vi "Main.vi"() -> ()   [LabVIEW 2025]
doc: "This template is for the Queued Message Handler design pattern.\n\nThe Event Handling Loop generates messages based on user interface actions.\n\nThe Message Handling Loop processes messages generated by the Event Handling Loop, or by other messages. The messages are string values, so new messages can be added easily to the Message Cases case structure in the Message Handling Loop. Each message cluster can also provide an optional value for Message Data, which is a variant that can be converted to whatever message-specific data is required."
uses:
  Example 01/Support/AC parameters--cluster.ctl
  Example 01/Support/IR parameters--cluster.ctl
  controls/UI Data.ctl
  controls/AC Params--cluster.ctl
  controls/IR Params--cluster.ctl
  controls/Acquisition Data.ctl
  controls/Settings--cluster.ctl
  controls/Step--numeric.ctl
  support/Message Queue/Enqueue Message (Single).vi
  <vilib>/Utility/error.llb/Error Cluster From Error Code.vi
  support/Message Queue/Enqueue Message (Array).vi
  <vilib>/ErrorRing/Error Ring.xnode
  support/Message Queue/Message Queue.lvlib
  support/User Event - Stop/User Event - Stop.lvlib
  <instrlib>/Chrome 19025/Chrome 19025.lvlib
panel:
  in  "Set IR":bool
  in  "Set AC":bool
  out "Conn?":bool caption="Connected?"
  in  "VISA resource name":refnum<visa-resource-name>
  in  "Stop Test":bool
  in  "Start Test":bool
  out "IR Resistance":dbl(graph)
  out "AC Test Current":dbl(graph)
  in  "IR Parameters":T1={"Voltage Level [V]"=500, "Hi Limit [ohm]"=30000000000.0, "Test Time [s] "=8.0, "Dwell Time [s]"=4.4, "Lo Limit [ohm]"=2500000.0, "Ramp Time [s] "=1.1, "Fall Time [s]"=2.2} {"Voltage Level [V]" min=50 max=1000 step=1 format="%.3p"; "Hi Limit [ohm]" min=0.0 max=50000000000000.0 step=100000.0 format="%.1p"; "Test Time [s]" min=0.0 max=999.0 step=0.1 format="%.1p"; "Dwell Time [s]" min=0.0 max=999.0 step=0.1 format="%.1p"; "Lo Limit [ohm]" min=100000.0 max=50000000000000.0 step=100000.0 format="%.1p"; "Ramp Time [s]" min=0.0 max=999.0 step=0.1 format="%.1p"; "Fall Time [s]" min=0.0 max=999.0 step=0.1 format="%.1p"}
  in  "AC Parameters":T2={"Voltage Level [V] "=1500, "Hi Limit [A]"=0.005, "Test Time [s] "=8.0, "Lo Limit [A]"=0.0001, "ARC Limit [A]"=0.005, "Ramp Time [s] "=1.1, "Fall Time [s]"=2.2} {"Voltage Level [V]" min=50 max=5000 step=1 format="%.3p"; "Hi Limit [A]" min=0.0001 max=0.03 step=1e-07 format="%.2p"; "Test Time [s]" min=0.0 max=999.0 step=0.1 format="%.1p"; "Lo Limit [A]" min=0.0 max=0.03 step=1e-07 format="%.2p"; "ARC Limit [A]" min=0.0 max=15.0 format="%.1p"; "Ramp Time [s]" min=0.0 max=999.0 step=0.1 format="%.1p"; "Fall Time [s]" min=0.0 max=999.0 step=0.1 format="%.1p"}
  out "Messages":string
  in  "Exit":bool
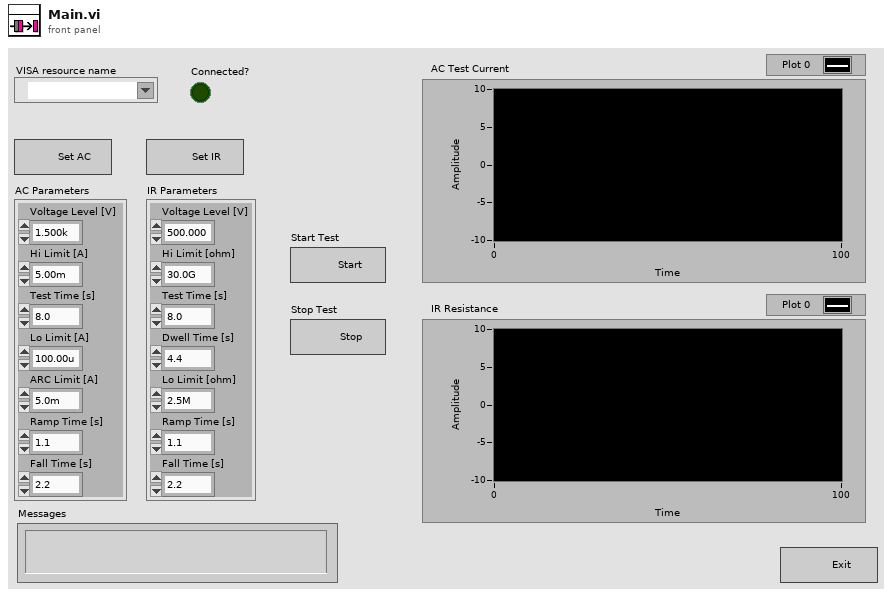
[diagram p1: front panel]
types:
  T1 = typedef "IR parameters--cluster.ctl" = cluster{"Voltage Level [V]":u16, "Hi Limit [ohm]":dbl, "Test Time [s] ":dbl, "Dwell Time [s]":dbl, "Lo Limit [ohm]":dbl, "Ramp Time [s] ":dbl, "Fall Time [s]":dbl}
  T2 = typedef "AC parameters--cluster.ctl" = cluster{"Voltage Level [V] ":u16, "Hi Limit [A]":dbl, "Test Time [s] ":dbl, "Lo Limit [A]":dbl, "ARC Limit [A]":dbl, "Ramp Time [s] ":dbl, "Fall Time [s]":dbl}
  T3 = typedef "UI Data.ctl" = cluster{"Connected?":bool, "Status":string, "Display Refnum":refnum<vi>, "Exit Refnum":refnum<vi>, "VISAName Refnum":refnum<vi>, "Settings":cluster{"VISA rsrc name":refnum<visa-resource-name>, "AC Parameters":T4, "IR Parameters":T5}}
  T4 = typedef "AC Params--cluster.ctl" = cluster{"Voltage Level [V] ":u16, "Hi Limit [A]":dbl, "Test Time [s] ":dbl, "Lo Limit [A]":dbl, "ARC Limit [A]":dbl, "Ramp Time [s] ":dbl, "Fall Time [s]":dbl}
  T5 = typedef "IR Params--cluster.ctl" = cluster{"Voltage Level [V]":u16, "Hi Limit [ohm]":dbl, "Test Time [s] ":dbl, "Dwell Time [s]":dbl, "Lo Limit [ohm]":dbl, "Ramp Time [s] ":dbl, "Fall Time [s]":dbl}
  T6 = typedef "Message Queue.lvlib/All Message Queues.ctl" = cluster{"UI":refnum<queue>, "Acquisition":refnum<queue>}
  T7 = cluster{"Baud Rate":u32, "Flow Control":u16, "Parity":u16, "Data Bits":u16}
  T8 = typedef "Settings--cluster.ctl" = cluster{"VISA rsrc name":refnum<visa-resource-name>, "AC Parameters":T4, "IR Parameters":T5}
  T9 = typedef "Acquisition Data.ctl" = cluster{"String <Replace Me>":string, "Numeric <Replace Me>":dbl, "Settings":cluster{"VISA rsrc name":refnum<visa-resource-name>, "AC Parameters":T4, "IR Parameters":T5}}
  T10 = typedef "Step--numeric.ctl" = u8
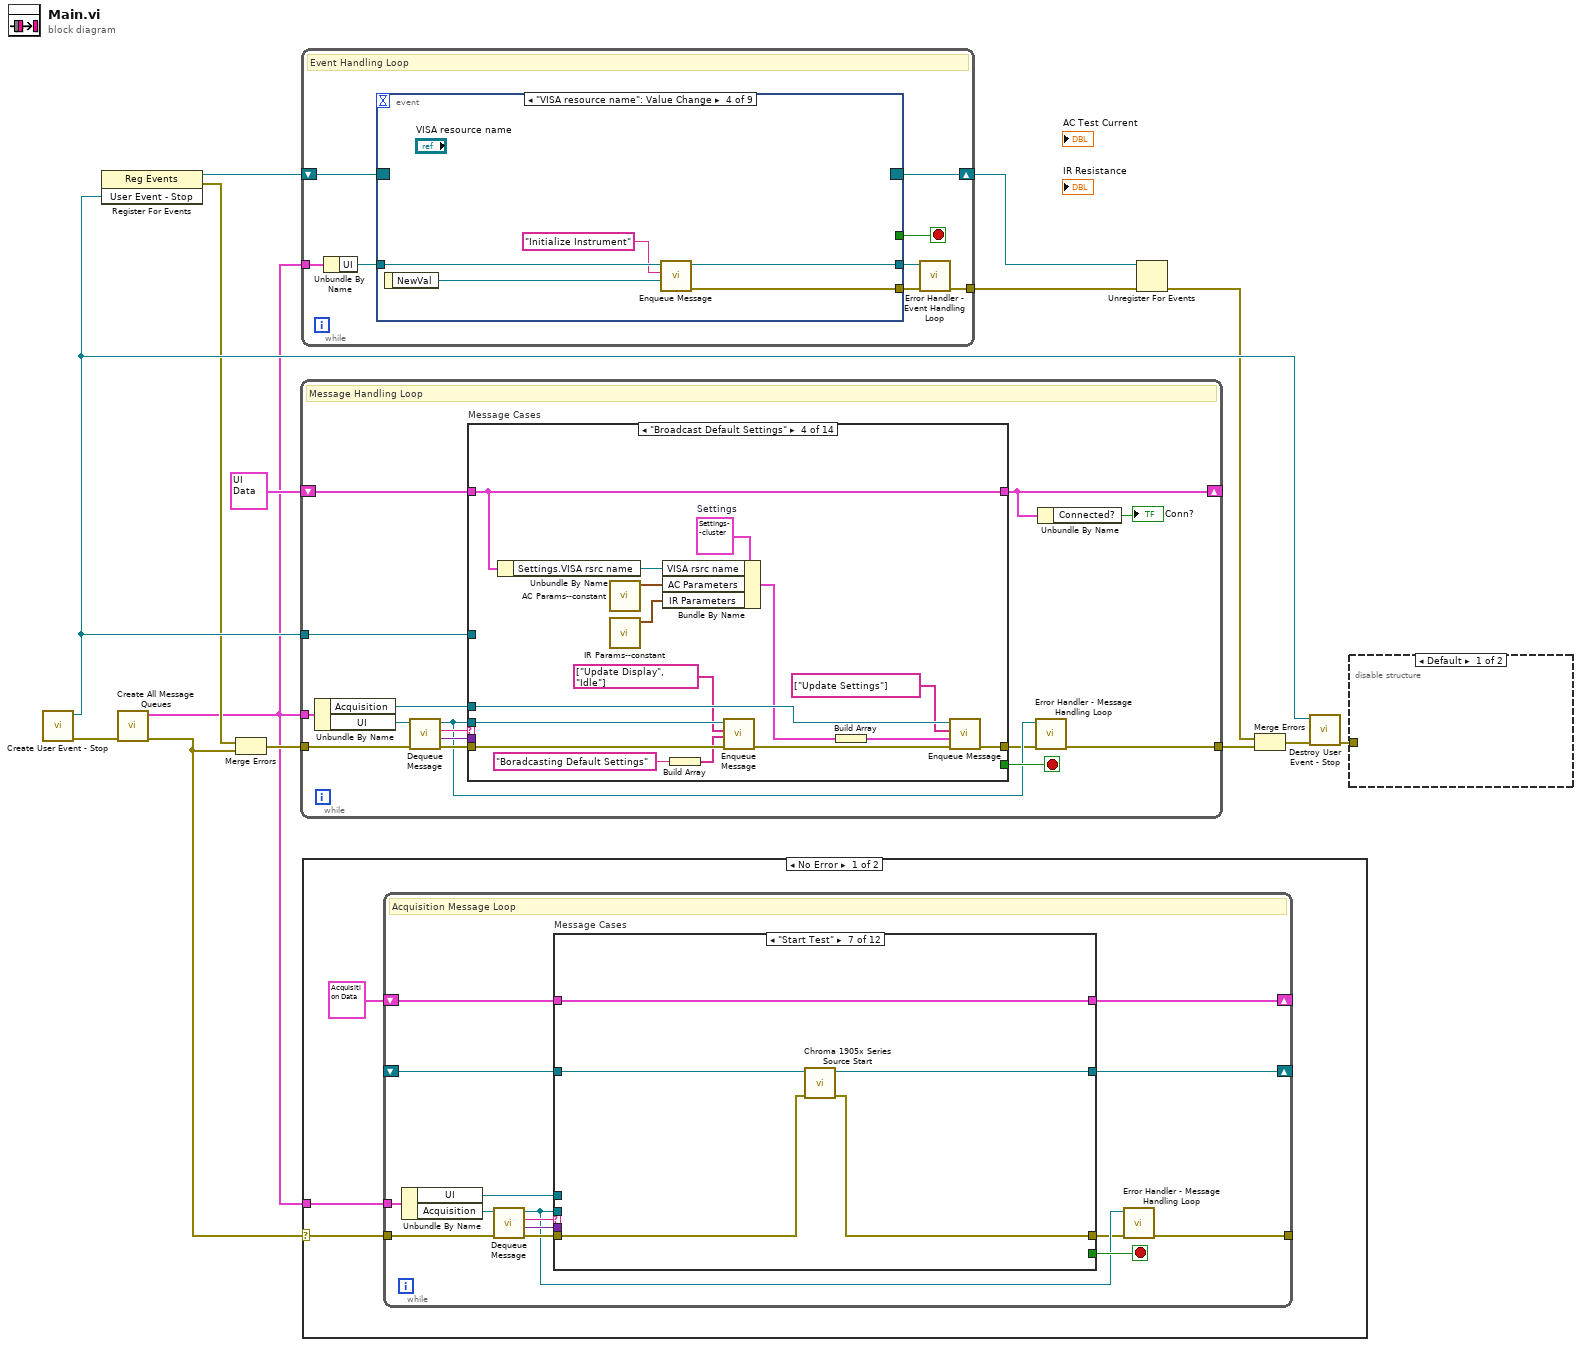
[diagram p0: block diagram]
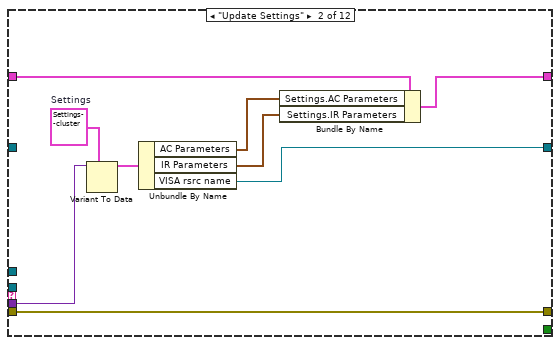
[diagram p3: hidden frame]
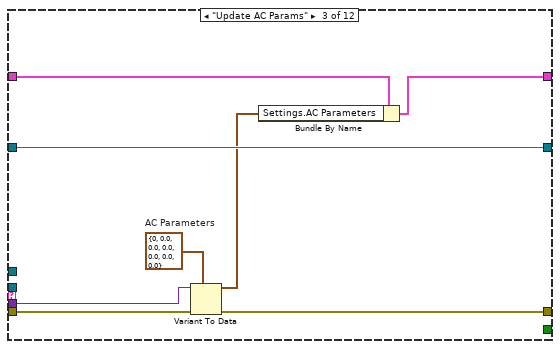
[diagram p4: hidden frame]
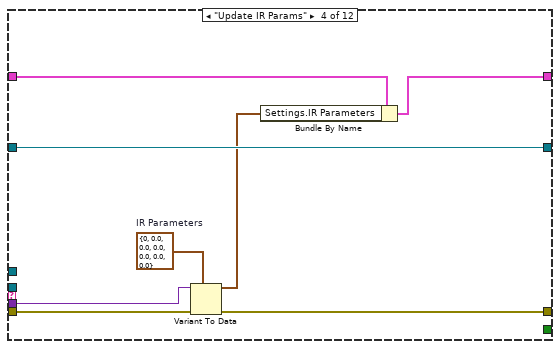
[diagram p5: hidden frame]
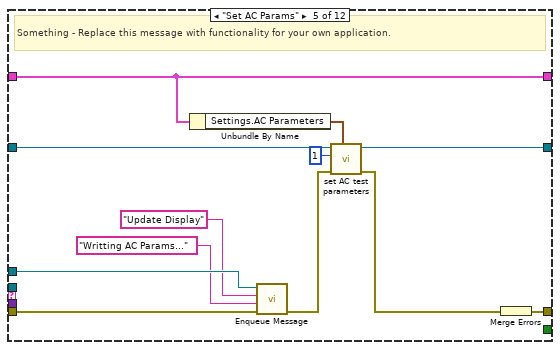
[diagram p6: hidden frame]
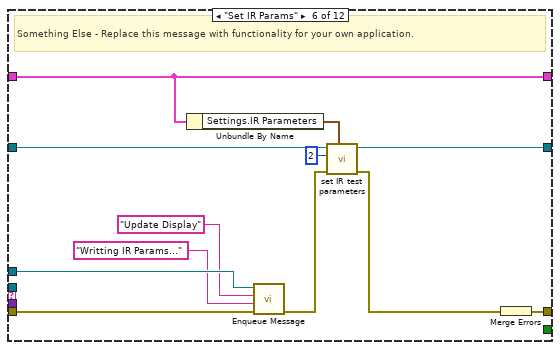
[diagram p7: hidden frame]
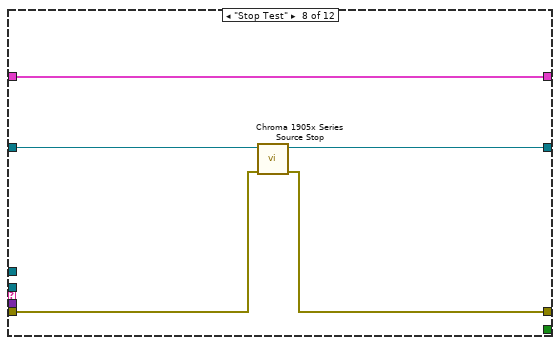
[diagram p8: hidden frame]
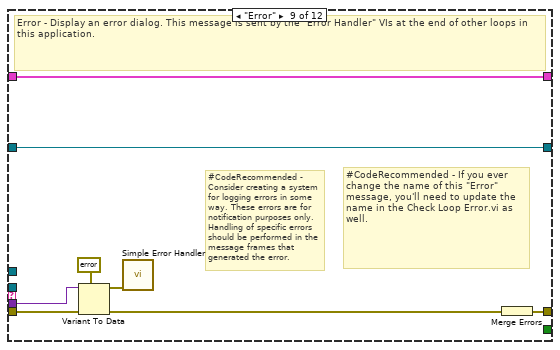
[diagram p9: hidden frame]
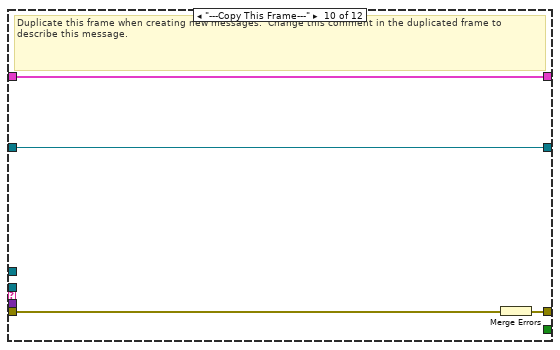
[diagram p10: hidden frame]
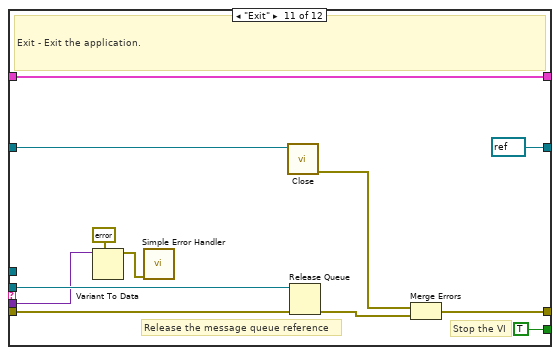
[diagram p11: hidden frame]
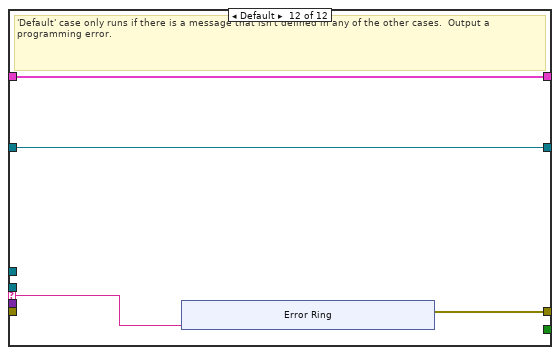
[diagram p12: hidden frame]
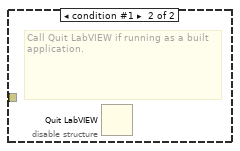
[diagram p14: hidden frame]
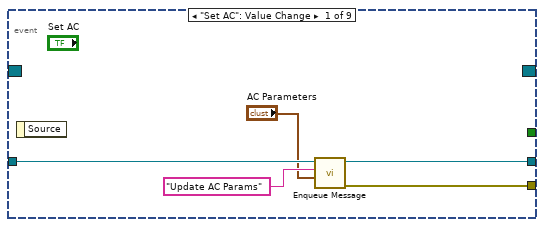
[diagram p15: hidden frame]
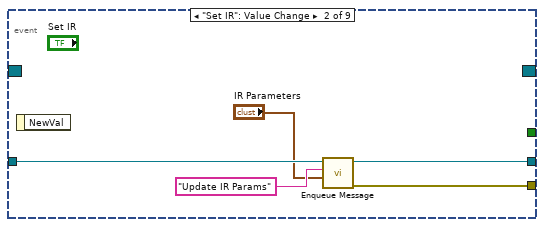
[diagram p16: hidden frame]
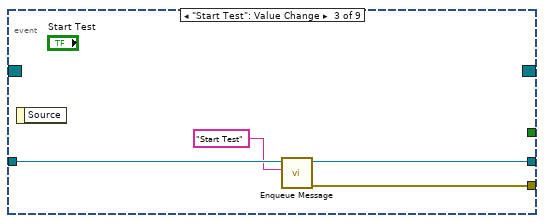
[diagram p17: hidden frame]
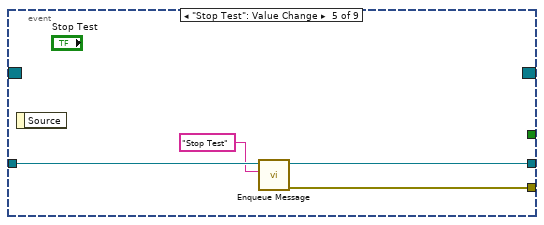
[diagram p18: hidden frame]
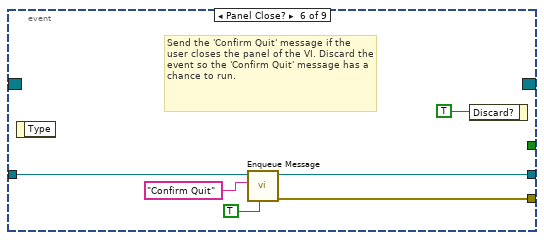
[diagram p19: hidden frame]
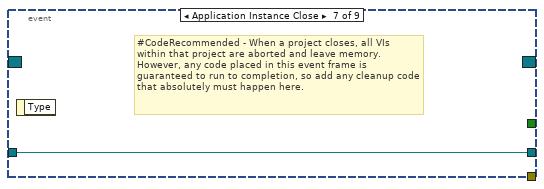
[diagram p20: hidden frame]
diagram:
  n1 = call "Create User Event - Stop.vi"() -> ("error out"=w11:errorcluster, "User Event - Stop"=w14:refnum<user-event>)  [unwired: 10 in]
  n2 = register-events(w14) -> (reference out=w4:refnum<event-registration>, error out=w13:errorcluster)  [unwired: 2 in]
  n3 = call "Create All Message Queues.vi"("error in (no error)"=w11) -> ("error out"=w2:errorcluster, "Message Queues out"=w1:T6)  [unwired: 9 in]
  n4 = Merge Errors(w13, w2) -> (w3:errorcluster)
  n5 = while {
    shift-right: [w17] -> _
    shift-left: T3 {"Connected?"=FALSE, "Status"="", "Display Refnum"=refnum, "Exit Refnum"=refnum, "VISAName Refnum"=refnum, "Settings"={"VISA rsrc name"="", "AC Parameters"={"Voltage Level [V] "=0, "Hi Limit [A]"=0.0, "Test Time [s] "=0.0, "Lo Limit [A]"=0.0, "ARC Limit [A]"=0.0, "Ramp Time [s] "=0.0, "Fall Time [s]"=0.0}, "IR Parameters"={"Voltage Level [V]"=0, "Hi Limit [ohm]"=0.0, "Test Time [s] "=0.0, "Dwell Time [s]"=0.0, "Lo Limit [ohm]"=0.0, "Ramp Time [s] "=0.0, "Fall Time [s]"=0.0}}} ("Data Cluster") -> [w29]
    tunnel: w14 -> [w27]
    tunnel: w3 -> [w26]
    tunnel: [w21] -> w12
    tunnel: w1 -> [w19]
    stop <- w28 stop-if-true
    # "Message Handling Loop"
    n6 = Unbundle By Name(w19) -> ("Acquisition"=w15:refnum<queue>, "UI"=w18:refnum<queue>)
    n7 = call "Dequeue Message.vi"("error in (no error)"=w26, "Message Queue"=w18) -> ("error out"=w25:errorcluster, "Message Data"=w23:variant, "Message"=w24:string, "dup Message Queue"=w22:refnum<queue>)  [unwired: 6 in]
    n8 = case "Message Cases" shown="\"Broadcast Default Settings\"" w24 {
      selector: w24 -> [_ _ _ _ _ _ _ _ _ _ _ _ _ w179]
      tunnel: w22 -> [w40 w45 w54 w80 w94 w105 w117 w124 _ _ w150 w161 w177 _]
      tunnel: w25 -> [w31 w44 w53 w82 w96 w114 w119 w132 w138 w147 w154 w156 w171 _]
      tunnel: [w39 w43 w55 w84 w100 w111 w122 w125 w139 w141 w152 w159 w174 w180] -> w20
      tunnel: w29 -> [w38 w47 w61 w78 w101 w112 w123 w130 w140 w146 w153 w160 w167 w181]
      tunnel: [w37 w46 w60 w78 w101 w112 w123 w130 w140 w146 w153 w160 w165 w181] -> w17
      tunnel: [_ _ _ _ _ _ _ _ _ _ _ _ TRUE _] -> w28
      tunnel: w23 -> [_ _ w50 _ w93 w106 _ _ w137 w145 _ _ w168 _]
      tunnel: w27 -> [_ _ _ _ _ _ _ _ _ _ _ _ w173 _]
      tunnel: w15 -> [_ _ _ w85 w99 w109 w121 w131 _ _ _ _ w178 _]
      frame "Initialize" {
        # "Initialize - All initialization work should take place in this message, since other loops can potentially enqueue messages that execute immediately after this one."
        n9 = control-ref of="VISA resource name"() -> (w30:refnum<vi>)
        n10 = control-ref of="Exit"() -> (w35:refnum<vi>)
        n11 = control-ref of="Display"() -> (w36:refnum<vi>)
        n12 = Bundle By Name(cluster=w38, "Display Refnum"=w36, "Exit Refnum"=w35, "VISAName Refnum"=w30) -> (w37:T3)
        n13 = Build Array("Initial Message" ("Initial Message")) -> (w32:string[])
        n14 = call-poly "Enqueue Message.vi"("error in (no error)"=w31, "Message Data Array"=w32, "Message Array"=string[] ["Update Display", "Get VISA Control Value"], "Message Queue"=w40) -> ("error out"=w39:errorcluster)  [unwired: 6 in, 1 out]
      }
      frame "Get VISA Control value" {
        n15 = Unbundle By Name(w47) -> ("VISAName Refnum"=w48:refnum<vi>)
        n16 = property class="VISAName"(reference=w48) -> ("Value"=w42:refnum<visa-resource-name>)  [unwired: 1 in, 2 out]
        n17 = Bundle By Name(cluster=w47, "Settings.VISA rsrc name"=w42) -> (w46:T3)
        n18 = call-poly "Enqueue Message.vi"("error in (no error)"=w44, "Message Data"=w42, "Message"="Initialize Instrument", "Message Queue"=w45) -> ("error out"=w43:errorcluster)  [unwired: 6 in, 1 out]
      }
      frame "Initialize Instrument" {
        n19 = call "Serial Params--constant.vi"() -> ("Serial Configuration"=w58:T7)  [unwired: 11 in]
        n20 = Variant To Data(error in=w53, type=refnum<visa-resource-name> refnum ("VISA resource name"), Variant=w50) -> (data=w49:refnum<visa-resource-name>, error out=w52:errorcluster)
        n21 = call <instrlib>:"Initialize.vi"("Serial Configuration"=w58, "error in (no error)"=w52, "Reset (True)"=FALSE, "VISA resource name"=w49) -> ("error out"=w56:errorcluster, "VISA resource name out"=w57:refnum<visa-resource-name>)  [unwired: 6 in]
        n22 = Not(x=w56) -> (.not. x?=w59:bool)
        n23 = case shown="No Error" w56 {
          selector: w56 -> [w66 w72]
          tunnel: [w65 w70] -> w55
          tunnel: w54 -> [w64 w69]
          frame No Error {
            n24 = call-poly "Enqueue Message.vi"("error in (no error)"=w66, "Message"="Broadcast Default Settings", "Message Queue"=w64) -> ("error out"=w65:errorcluster)  [unwired: 7 in, 1 out]
          }
          frame Error {
            n25 = call <vilib>:"Clear Errors.vi"("error in (no error)"=w72) -> ("error out"=w71:errorcluster)  [unwired: 5 in, 1 out]
            n26 = call-poly "Enqueue Message.vi"("error in (no error)"=w71, "Message Data"="Connection Error. Update VISA reference number to retry connection.", "Message"="Update Display", "Message Queue"=w69) -> ("error out"=w70:errorcluster)  [unwired: 6 in, 1 out]
          }
        }
        n27 = Bundle By Name(cluster=w61, "Settings.VISA rsrc name"=w57, "Connected?"=w59) -> (w60:T3)
      }
      frame "Broadcast Default Settings" {
        w86 = T8 {"VISA rsrc name"="", "AC Parameters"={"Voltage Level [V] "=0, "Hi Limit [A]"=0.0, "Test Time [s] "=0.0, "Lo Limit [A]"=0.0, "ARC Limit [A]"=0.0, "Ramp Time [s] "=0.0, "Fall Time [s]"=0.0}, "IR Parameters"={"Voltage Level [V]"=0, "Hi Limit [ohm]"=0.0, "Test Time [s] "=0.0, "Dwell Time [s]"=0.0, "Lo Limit [ohm]"=0.0, "Ramp Time [s] "=0.0, "Fall Time [s]"=0.0}}  # Settings
        n28 = Unbundle By Name(w78) -> ("Settings.VISA rsrc name"=w77:refnum<visa-resource-name>)
        n29 = call "AC Params--constant.vi"() -> ("AC Parameters"=w88:T4)  [unwired: 11 in]
        n30 = call "IR Params--constant.vi"() -> ("IR Parameters"=w87:T5)  [unwired: 11 in]
        n31 = Bundle By Name(cluster=w86, "VISA rsrc name"=w77, "AC Parameters"=w88, "IR Parameters"=w87) -> (w83:T8)
        n32 = Build Array("Boradcasting Default Settings") -> (w73:string[])
        n33 = call-poly "Enqueue Message.vi"("error in (no error)"=w82, "Message Data Array"=w73, "Message Array"=string[] ["Update Display", "Idle"], "Message Queue"=w80) -> ("error out"=w81:errorcluster)  [unwired: 6 in, 1 out]
        n34 = Build Array(w83) -> (w75:T8[])
        n35 = call-poly "Enqueue Message.vi"("error in (no error)"=w81, "Message Data Array"=w75, "Message Array"=string[] ["Update Settings"], "Message Queue"=w85) -> ("error out"=w84:errorcluster)  [unwired: 6 in, 1 out]
      }
      frame "Update AC Params" {
        # "Something - Replace this message with functionality for your own application."
        n36 = Build Array("Updating AC Params") -> (w89:string[])
        n37 = call-poly "Enqueue Message.vi"("error in (no error)"=w96, "Message Data Array"=w89, "Message Array"=string[] ["Update Display", "Idle"], "Message Queue"=w94) -> ("error out"=w95:errorcluster)  [unwired: 6 in, 1 out]
        n38 = Build Array(w93) -> (w92:variant[])
        n39 = call-poly "Enqueue Message.vi"("error in (no error)"=w95, "Message Data Array"=w92, "Message Array"=string[] ["Update AC Params", "Set AC Params"], "Message Queue"=w99) -> ("error out"=w98:errorcluster)  [unwired: 6 in, 1 out]
        n40 = Merge Errors(w98) -> (w100:errorcluster)
      }
      frame "Update IR Params" {
        # "Something Else - Replace this message with functionality for your own application."
        n41 = Build Array("Updating IR Params") -> (w102:string[])
        n42 = call-poly "Enqueue Message.vi"("error in (no error)"=w114, "Message Data Array"=w102, "Message Array"=string[] ["Update Display", "Idle"], "Message Queue"=w105) -> ("error out"=w113:errorcluster)  [unwired: 6 in, 1 out]
        n43 = Build Array(w106) -> (w108:variant[])
        n44 = call-poly "Enqueue Message.vi"("error in (no error)"=w113, "Message Data Array"=w108, "Message Array"=string[] ["Update IR Params", "Set IR Params"], "Message Queue"=w109) -> ("error out"=w110:errorcluster)  [unwired: 6 in, 1 out]
        n45 = Merge Errors(w110) -> (w111:errorcluster)
      }
      frame "Start Test" {
        n46 = call-poly "Enqueue Message.vi"("error in (no error)"=w119, "Message Data"="Starting Test..." ("Message"), "Message"="Update Display", "Message Queue"=w117) -> ("error out"=w118:errorcluster)  [unwired: 6 in, 1 out]
        n47 = call-poly "Enqueue Message.vi"("error in (no error)"=w118, "Message"="Start Test", "Message Queue"=w121) -> ("error out"=w122:errorcluster)  [unwired: 7 in, 1 out]
      }
      frame "Stop Test" {
        n48 = call-poly "Enqueue Message.vi"("error in (no error)"=w132, "Message Data"="Stopping Test..." ("Message"), "Message"="Update Display", "Message Queue"=w124) -> ("error out"=w128:errorcluster)  [unwired: 6 in, 1 out]
        n49 = call-poly "Enqueue Message.vi"("error in (no error)"=w128, "Message"="Stop Test", "Message Queue"=w131) -> ("error out"=w125:errorcluster)  [unwired: 7 in, 1 out]
      }
      frame "Update Display" {
        # "#CodeRecommended - If you wish to decouple the Message Handling Loop from your user interface, consider creating User Events (like the \"Stop\" event in this VI) to message the Event Handling Loop whenever the user interface needs updating."
        # "Update Display - Convert the message data to a string to display in the Data Display indicator."
        n50 = Variant To Data(error in=w138, type="", Variant=w137) -> (data=→"Messages":string, error out=w135:errorcluster)
        n51 = Wait (ms)(milliseconds to wait=u32 250) -> ()  [unwired: 1 out]
        n52 = Merge Errors(w135) -> (w139:errorcluster)
      }
      frame "Error" {
        # "#CodeRecommended - If you ever change the name of this \"Error\" message, you'll need to update the name in the Check Loop Error.vi as well."
        # "#CodeRecommended - Consider creating a system for logging errors in some way. These errors are for notification purposes only. Handling of specific errors should be performed in the message frames that generated the error."
        # "Error - Display an error dialog. This message is sent by the \"Error Handler\" VIs at the end of other loops in this application."
        n53 = Variant To Data(error in=w147, type=errorcluster {"status"=FALSE, "code"=0, "source"=""} ("error constant"), Variant=w145) -> (data=w143:errorcluster, error out=w142:errorcluster)
        n54 = call <vilib>:"Simple Error Handler.vi"("error in (no error)"=w143) -> ()  [unwired: 4 in, 5 out]
        n55 = Merge Errors(w142) -> (w141:errorcluster)
      }
      frame "Confirm Quit" {
        # "#CodeNeeded - If you want to provide an \"Are you sure\" dialog (or some other notification) before the application exits, place that code here. This message is typically sent from a Panel Close? event."
        # "Confirm Quit - Message that can confirm whether or not the user wants to exit the application."
        n56 = call-poly "Enqueue Message.vi"("Priority Message? (F)"=TRUE, "error in (no error)"=w154, "Message"="Exit", "Message Queue"=w150) -> ("error out"=w151:errorcluster)  [unwired: 6 in, 1 out]
        n57 = Merge Errors(w151) -> (w152:errorcluster)
      }
      frame "Idle" {
        n58 = call-poly "Enqueue Message.vi"("error in (no error)"=w156, "Message Data"="Ready...", "Message"="Update Display", "Message Queue"=w161) -> ("error out"=w155:errorcluster)  [unwired: 6 in, 1 out]
        n59 = Merge Errors(w155) -> (w159:errorcluster)
      }
      frame "Exit" {
        # "Stop the VI"
        # "Release the message queue reference"
        # "Exit - Exit the application."
        n60 = Variant To Data(type=errorcluster {"status"=FALSE, "code"=0, "source"=""} ("error constant"), Variant=w168) -> (data=w169:errorcluster)  [unwired: 1 in, 1 out]
        n61 = call <vilib>:"Simple Error Handler.vi"("error in (no error)"=w169) -> ()  [unwired: 4 in, 5 out]
        n62 = call-poly "Enqueue Message.vi"("Priority Message? (F)"=TRUE, "Message"="Exit", "Message Queue"=w178) -> ("error out"=w162:errorcluster)  [unwired: 7 in, 1 out]
        n63 = call "Fire User Event - Stop.vi"("User Event - Stop"=w173) -> ("error out"=w172:errorcluster)  [unwired: 10 in]
        n64 = Release Queue(queue=w177, error in (no error)=w171) -> (error out=w175:errorcluster)  [unwired: 1 in, 2 out]
        n65 = Bundle By Name(cluster=w167, "Connected?"=FALSE) -> (w165:T3)
        n66 = Merge Errors(w162, w172, w175) -> (w174:errorcluster)
      }
      frame Default {
        # "'Default' case only runs if there is a message that isn't defined in any of the other cases.  Output a programming error."
        n67 = xnode "Error Ring"("parameter 0"=w179) -> ("error out"=w180:errorcluster)
      }
    }
    n68 = call "Error Handler - Message Handling Loop.vi"("error in (no error)"=w20, "Message Queue"=w22) -> ("dup error in"=w21:errorcluster)  [unwired: 8 in, 1 out]
    n69 = Unbundle By Name(w17) -> ("Connected?"=→"Conn?":bool)
  }
  n70 = while {
    shift-right: [w195] -> w8
    shift-left: w4 -> [w196]
    tunnel: [w191] -> w5
    tunnel: w1 -> [w190]
    stop <- w193 stop-if-true
    # "Event Handling Loop"
    n71 = Unbundle By Name(w190) -> ("UI"=w189:refnum<queue>)
    n72 = event shown="[3] \"VISA resource name\": Value Change" {
      selector: w196 -> [_ _ _ _ _ _ _ _ _]
      dyn-events: [_ _ _ _ _ _ _ _ _] -> w195
      timeout: _ -> [_ _ _ _ _ _ _ _ _]
      tunnel: [_ _ _ _ _ _ _ _ TRUE ("Discard?")] -> w193
      tunnel: w189 -> [w201 w206 w210 w215 w219 w224 w226 w231 w234]
      tunnel: [w198 w203 w208 w213 w217 w223 _ w230 _] -> w194
      tunnel: [w200 w205 w209 w214 w218 w222 w226 w229 w234] -> w192
      event "Set AC": Value Change {
        n73 = event-data() -> ()  [unwired: 1 in, 1 out]
        n74 = call-poly "Enqueue Message.vi"("Message Data"="AC Parameters", "Message"="Update AC Params", "Message Queue"=w201) -> ("error out"=w198:errorcluster, "dup Message Queue"=w200:refnum<queue>)  [unwired: 7 in]
      }
      event "Set IR": Value Change {
        n75 = event-data() -> ()  [unwired: 1 in, 1 out]
        n76 = call-poly "Enqueue Message.vi"("Message Data"="IR Parameters", "Message"="Update IR Params", "Message Queue"=w206) -> ("error out"=w203:errorcluster, "dup Message Queue"=w205:refnum<queue>)  [unwired: 7 in]
      }
      event "Start Test": Value Change {
        n77 = event-data() -> ()  [unwired: 1 in, 1 out]
        n78 = call-poly "Enqueue Message.vi"("Message"="Start Test", "Message Queue"=w210) -> ("error out"=w208:errorcluster, "dup Message Queue"=w209:refnum<queue>)  [unwired: 8 in]
      }
      event "VISA resource name": Value Change {
        n79 = event-data() -> ("NewVal"=w212:refnum<visa-resource-name>)  [unwired: 1 in]
        n80 = call-poly "Enqueue Message.vi"("Message Data"=w212, "Message"="Initialize Instrument", "Message Queue"=w215) -> ("error out"=w213:errorcluster, "dup Message Queue"=w214:refnum<queue>)  [unwired: 7 in]
      }
      event "Stop Test": Value Change {
        n81 = event-data() -> ()  [unwired: 1 in, 1 out]
        n82 = call-poly "Enqueue Message.vi"("Message"="Stop Test", "Message Queue"=w219) -> ("error out"=w217:errorcluster, "dup Message Queue"=w218:refnum<queue>)  [unwired: 8 in]
      }
      event Panel Close? {
        # "Send the 'Confirm Quit' message if the user closes the panel of the VI. Discard the event so the 'Confirm Quit' message has a chance to run."
        n83 = event-data() -> ()  [unwired: 1 in, 1 out]
        n84 = call-poly "Enqueue Message.vi"("Priority Message? (F)"=TRUE, "Message"="Confirm Quit", "Message Queue"=w224) -> ("error out"=w223:errorcluster, "dup Message Queue"=w222:refnum<queue>)  [unwired: 7 in]
        n85 = event-data("Discard?"=TRUE) -> ()  [unwired: 1 in, 1 out]
      }
      event Application Instance Close {
        # "#CodeRecommended - When a project closes, all VIs within that project are aborted and leave memory. However, any code placed in this event frame is guaranteed to run to completion, so add any cleanup code that absolutely must happen here."
        n86 = event-data() -> ()  [unwired: 1 in, 1 out]
      }
      event "Exit": Value Change {
        n87 = event-data() -> ()  [unwired: 1 in, 1 out]
        n88 = call-poly "Enqueue Message.vi"("Priority Message? (F)"=TRUE, "Message"="Exit", "Message Queue"=w231) -> ("error out"=w230:errorcluster, "dup Message Queue"=w229:refnum<queue>)  [unwired: 7 in]
      }
      event User Event {
        # "The Message Handling Loop processed an \"Exit\" message, which fired this event to stop the Event Handling Loop."
        n89 = event-data() -> ()  [unwired: 1 in, 1 out]
        n90 = local write "Messages"("\"Exit\" button pressed" ("VI Stopped")) -> ()
      }
    }
    n91 = call "Error Handler - Event Handling Loop.vi"("error in (no error)"=w194, "Message Queue"=w192) -> ("dup error in"=w191:errorcluster)  [unwired: 8 in, 1 out]
  }
  n92 = case shown="No Error" w2 {
    selector: w2 -> [w237 _]
    tunnel: w1 -> [w236 _]
    frame No Error {
      n93 = while {
        shift-right: [w243] -> _
        shift-left: T9 {"String <Replace Me>"="", "Numeric <Replace Me>"=0.0, "Settings"={"VISA rsrc name"="", "AC Parameters"={"Voltage Level [V] "=0, "Hi Limit [A]"=0.0, "Test Time [s] "=0.0, "Lo Limit [A]"=0.0, "ARC Limit [A]"=0.0, "Ramp Time [s] "=0.0, "Fall Time [s]"=0.0}, "IR Parameters"={"Voltage Level [V]"=0, "Hi Limit [ohm]"=0.0, "Test Time [s] "=0.0, "Dwell Time [s]"=0.0, "Lo Limit [ohm]"=0.0, "Ramp Time [s] "=0.0, "Fall Time [s]"=0.0}}} ("Acq Data") -> [w252]
        tunnel: w237 -> [w250]
        tunnel: [w245] -> _
        tunnel: w236 -> [w242]
        shift-right: [w240] -> _
        shift-left: _ -> [w239]
        stop <- w251 stop-if-true
        # "Acquisition Message Loop"
        n94 = Unbundle By Name(w242) -> ("UI"=w238:refnum<queue>, "Acquisition"=w241:refnum<queue>)
        n95 = call "Dequeue Message.vi"("error in (no error)"=w250, "Message Queue"=w241) -> ("error out"=w249:errorcluster, "Message Data"=w247:variant, "Message"=w248:string, "dup Message Queue"=w246:refnum<queue>)  [unwired: 6 in]
        n96 = case "Message Cases" shown="\"Start Test\"" w248 {
          selector: w248 -> [_ _ _ _ _ _ _ _ _ _ _ w340]
          tunnel: w246 -> [_ _ _ _ _ _ _ _ _ _ w338 _]
          tunnel: w249 -> [w253 w256 w269 w277 w283 w295 w306 w312 w322 w326 w334 _]
          tunnel: [w253 w256 w268 w276 w291 w303 w305 w311 w316 w324 w335 w341] -> w244
          tunnel: w252 -> [w254 w260 w271 w279 w288 w299 w309 w314 w321 w325 w327 w342]
          tunnel: [w254 w257 w270 w278 w288 w299 w309 w314 w321 w325 w327 w342] -> w243
          tunnel: [_ _ _ _ _ _ _ _ _ _ TRUE _] -> w251
          tunnel: w247 -> [_ w263 w267 w275 _ _ _ _ w320 _ w331 _]
          tunnel: [w255 w261 w272 w280 w290 w302 w307 w313 w315 w323 refnum<visa-resource-name> refnum ("VISA resource name") w339] -> w240
          tunnel: w239 -> [w255 _ w272 w280 w286 w298 w308 w310 w315 w323 w329 w339]
          tunnel: w238 -> [_ _ _ _ w292 w304 _ _ _ _ _ _]
          frame "Initialize" {
            # "Initialize - All initialization work should take place in this message, since other loops can potentially enqueue messages that execute immediately after this one."
          }
          frame "Update Settings" {
            w264 = T8 {"VISA rsrc name"="", "AC Parameters"={"Voltage Level [V] "=0, "Hi Limit [A]"=0.0, "Test Time [s] "=0.0, "Lo Limit [A]"=0.0, "ARC Limit [A]"=0.0, "Ramp Time [s] "=0.0, "Fall Time [s]"=0.0}, "IR Parameters"={"Voltage Level [V]"=0, "Hi Limit [ohm]"=0.0, "Test Time [s] "=0.0, "Dwell Time [s]"=0.0, "Lo Limit [ohm]"=0.0, "Ramp Time [s] "=0.0, "Fall Time [s]"=0.0}}  # Settings
            n97 = Variant To Data(type=w264, Variant=w263) -> (data=w262:T8)  [unwired: 1 in, 1 out]
            n98 = Unbundle By Name(w262) -> ("AC Parameters"=w259:T4, "IR Parameters"=w258:T5, "VISA rsrc name"=w261:refnum<visa-resource-name>)
            n99 = Bundle By Name(cluster=w260, "Settings.AC Parameters"=w259, "Settings.IR Parameters"=w258) -> (w257:T9)
          }
          frame "Update AC Params" {
            w266 = T4 {"Voltage Level [V] "=0, "Hi Limit [A]"=0.0, "Test Time [s] "=0.0, "Lo Limit [A]"=0.0, "ARC Limit [A]"=0.0, "Ramp Time [s] "=0.0, "Fall Time [s]"=0.0}  # AC Parameters
            n100 = Variant To Data(error in=w269, type=w266, Variant=w267) -> (data=w265:T4, error out=w268:errorcluster)
            n101 = Bundle By Name(cluster=w271, "Settings.AC Parameters"=w265) -> (w270:T9)
          }
          frame "Update IR Params" {
            w274 = T5 {"Voltage Level [V]"=0, "Hi Limit [ohm]"=0.0, "Test Time [s] "=0.0, "Dwell Time [s]"=0.0, "Lo Limit [ohm]"=0.0, "Ramp Time [s] "=0.0, "Fall Time [s]"=0.0}  # IR Parameters
            n102 = Variant To Data(error in=w277, type=w274, Variant=w275) -> (data=w273:T5, error out=w276:errorcluster)
            n103 = Bundle By Name(cluster=w279, "Settings.IR Parameters"=w273) -> (w278:T9)
          }
          frame "Set AC Params" {
            # "Something - Replace this message with functionality for your own application."
            n104 = Unbundle By Name(w288) -> ("Settings.AC Parameters"=w287:T4)
            n105 = call-poly "Enqueue Message.vi"("error in (no error)"=w283, "Message Data"="Writting AC Params...", "Message"="Update Display", "Message Queue"=w292) -> ("error out"=w284:errorcluster)  [unwired: 6 in, 1 out]
            n106 = call "set AC test parameters.vi"("AC Parameters"=w287, "error in (no error)"=w284, "Step"=T10 1, "VISA Refnum in"=w286) -> ("error out"=w289:errorcluster, "VISA Refnum out"=w290:refnum<visa-resource-name>)  [unwired: 6 in]
            n107 = Merge Errors(w289) -> (w291:errorcluster)
          }
          frame "Set IR Params" {
            # "Something Else - Replace this message with functionality for your own application."
            n108 = Unbundle By Name(w299) -> ("Settings.IR Parameters"=w300:T5)
            n109 = call-poly "Enqueue Message.vi"("error in (no error)"=w295, "Message Data"="Writting IR Params...", "Message"="Update Display", "Message Queue"=w304) -> ("error out"=w294:errorcluster)  [unwired: 6 in, 1 out]
            n110 = call "set IR test parameters.vi"("IR Parameters"=w300, "error in (no error)"=w294, "Step"=T10 2, "VISA Refnum in"=w298) -> ("error out"=w301:errorcluster, "VISA Refnum out"=w302:refnum<visa-resource-name>)  [unwired: 6 in]
            n111 = Merge Errors(w301) -> (w303:errorcluster)
          }
          frame "Start Test" {
            n112 = call "Chroma 1905x Series Source Start.vi"("error in (no error)"=w306, "VISA resource name"=w308) -> ("error out"=w305:errorcluster, "VISA resource name out"=w307:refnum<visa-resource-name>)  [unwired: 8 in]
          }
          frame "Stop Test" {
            n113 = call "Chroma 1905x Series Source Stop.vi"("error in (no error)"=w312, "VISA resource name"=w310) -> ("error out"=w311:errorcluster, "VISA resource name out"=w313:refnum<visa-resource-name>)  [unwired: 8 in]
          }
          frame "Error" {
            # "#CodeRecommended - If you ever change the name of this \"Error\" message, you'll need to update the name in the Check Loop Error.vi as well."
            # "#CodeRecommended - Consider creating a system for logging errors in some way. These errors are for notification purposes only. Handling of specific errors should be performed in the message frames that generated the error."
            # "Error - Display an error dialog. This message is sent by the \"Error Handler\" VIs at the end of other loops in this application."
            n114 = Variant To Data(error in=w322, type=errorcluster {"status"=FALSE, "code"=0, "source"=""} ("error constant"), Variant=w320) -> (data=w318:errorcluster, error out=w317:errorcluster)
            n115 = call <vilib>:"Simple Error Handler.vi"("error in (no error)"=w318) -> ()  [unwired: 4 in, 5 out]
            n116 = Merge Errors(w317) -> (w316:errorcluster)
          }
          frame "---Copy This Frame---" {
            # "Duplicate this frame when creating new messages.  Change this comment in the duplicated frame to describe this message."
            n117 = Merge Errors(w326) -> (w324:errorcluster)
          }
          frame "Exit" {
            # "Stop the VI"
            # "Release the message queue reference"
            # "Exit - Exit the application."
            n118 = Variant To Data(type=errorcluster {"status"=FALSE, "code"=0, "source"=""} ("error constant"), Variant=w331) -> (data=w332:errorcluster)  [unwired: 1 in, 1 out]
            n119 = call <vilib>:"Simple Error Handler.vi"("error in (no error)"=w332) -> ()  [unwired: 4 in, 5 out]
            n120 = call <instrlib>:"Close.vi"("VISA resource name"=w329) -> ("error out"=w328:errorcluster)  [unwired: 10 in]
            n121 = Release Queue(queue=w338, error in (no error)=w334) -> (error out=w336:errorcluster)  [unwired: 1 in, 2 out]
            n122 = Merge Errors(w328, w336) -> (w335:errorcluster)
          }
          frame Default {
            # "'Default' case only runs if there is a message that isn't defined in any of the other cases.  Output a programming error."
            n123 = xnode "Error Ring"("parameter 0"=w340) -> ("error out"=w341:errorcluster)
          }
        }
        n124 = call "Error Handler - Message Handling Loop.vi"("error in (no error)"=w244, "Message Queue"=w246) -> ("dup error in"=w245:errorcluster)  [unwired: 8 in, 1 out]
      }
    }
    frame Error {
    }
  }
  n125 = Unregister For Events(event registration refnum=w8, error in=w5) -> (error out=w9:errorcluster)
  n126 = Merge Errors(w9, w12) -> (w10:errorcluster)
  n127 = call "Destroy User Event - Stop.vi"("error in (no error)"=w10, "User Event - Stop"=w14) -> ("error out"=w6:errorcluster)  [unwired: 9 in]
  n128 = disable-structure shown="Default" {
    disable-tunnel: w6 -> [_ _]
    frame condition #0 (active) {
    }
    frame condition #1 {
      # "Call Quit LabVIEW if running as a built application."
      n129 = Quit LabVIEW() -> ()  [unwired: 1 in]
    }
  }
